vi "Generate Random Delay.vi"(0 "Min (ms)":dbl=200.0, 5 "Max (ms)":dbl=200.0, 7 "Prob":dbl=0.1, 11 "error in (no error)":errorcluster) -> (8 "millisecond timer value":u32, 15 "error out":errorcluster)   [LabVIEW 2015]
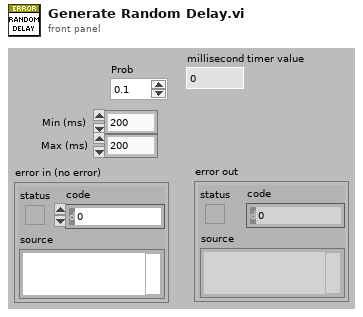
[diagram p1: front panel]
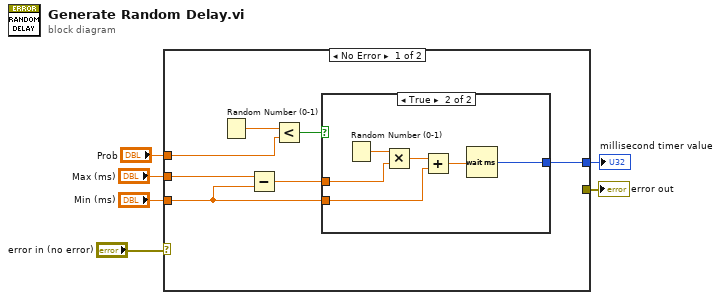
[diagram p0: block diagram]
diagram:
  n1 = case shown="No Error" "error in (no error)" {
    selector: "error in (no error)" -> [_ w20]
    tunnel: [_ w20] -> w5
    tunnel: "Prob" -> [w11 _]
    tunnel: "Max (ms)" -> [w10 _]
    tunnel: "Min (ms)" -> [w8 _]
    tunnel: [w7 _] -> w1
    frame No Error {
      n2 = Random Number (0-1)() -> (number: 0 to 1=w13:dbl)
      n3 = Subtract(x=w10, y=w8) -> (x-y=w9:dbl)
      n4 = Less?(x=w13, y=w11) -> (x < y?=w12:bool)
      n5 = case shown="True" w12 {
        tunnel: w9 -> [_ w18]
        tunnel: w8 -> [_ w16]
        tunnel: [_ w14] -> w7
        frame False {
        }
        frame True {
          n6 = Random Number (0-1)() -> (number: 0 to 1=w19:dbl)
          n7 = Multiply(x=w19, y=w18) -> (x*y=w17:dbl)
          n8 = Add(x=w17, y=w16) -> (x+y=w15:dbl)
          n9 = Wait (ms)(milliseconds to wait=w15) -> (millisecond timer value=w14:u32)
        }
      }
    }
    frame Error {
    }
  }
  "error out" <- w5
  "millisecond timer value" <- w1
